vi "AB_Engine_Is_Instance_VI.vi"(11 "File":T2) -> (3 "Is Instance VI?":bool)   [LabVIEW 2020]
uses:
  <vilib>/Utility/lvfile.llb/LVFileType.ctl
  <vilib>/Utility/lvfile.llb/NI_FileType.lvlib
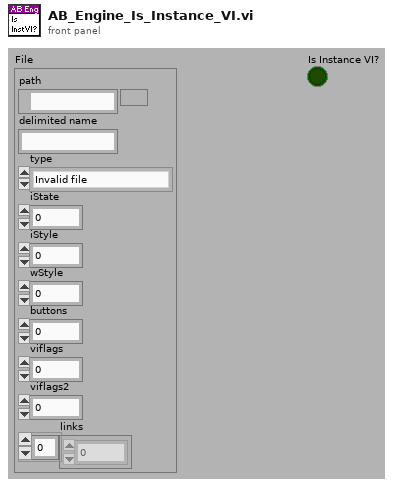
[diagram p1: front panel]
types:
  T1 = typedef "NI_FileType.lvlib/LVFileType.ctl" = enum32{"Invalid file", "Unknown type", "Instrument", "Control", "Polymorphic VI", "Project", "Library", "LVClass", "XControl", "XNode", "Shared library", ".NET assembly", "ActiveX interface", "CIN", "Run-time menu", "Palette menu", "Help file", "LLB", "XNode Edit Dependency", "Class Private Data Control", "Statechart", "MathScript .m file", "Ladder Diagram", "LVLibp", "XNode Build Dependency"}
  T2 = cluster{"path":path, "delimited name":string, "type":T1, "iState":u32, "iStyle":u16, "wStyle":u16, "buttons":u16, "viflags":u32, "viflags2":u32, "links":u32[]}
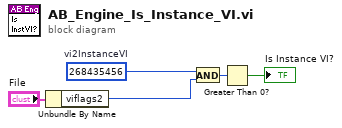
[diagram p0: block diagram]
diagram:
  w3 = u32 268435456  # vi2InstanceVI
  n1 = Unbundle By Name("File") -> ("viflags2"=w4:u32)
  n2 = And(x=w3, y=w4) -> (x .and. y?=w2:u32)
  n3 = Greater Than 0?(x=w2) -> (x > 0?=→"Is Instance VI?":bool)
